vi "Start Stop graph.vi"(8 "error in (no error)":errorcluster, 10 "Start/Stop":bool, 11 "F Generator in":refnum<class "F Generator.lvclass">) -> (0 "error out":errorcluster, 3 "F Generator out":refnum<class "F Generator.lvclass">)   [LabVIEW 2020, in "F Generator.lvlib" / "F Generator.lvclass"]
uses:
  F Generator.lvclass
  F Generator.lvclass/F Generator.ctl
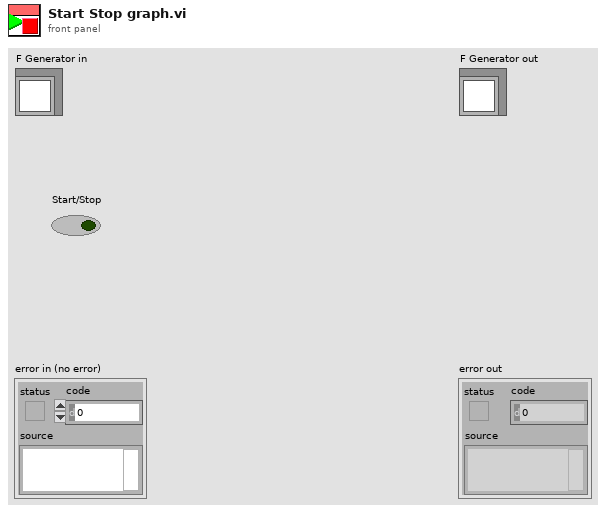
[diagram p1: front panel]
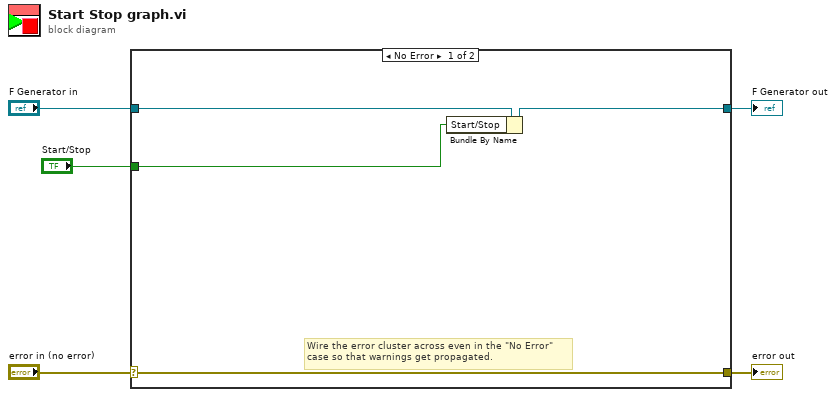
[diagram p0: block diagram]
diagram:
  n1 = case shown="No Error" "error in (no error)" {
    selector: "error in (no error)" -> [w8 w11]
    tunnel: [w8 w11] -> w4
    tunnel: [w7 w10] -> w2
    tunnel: "F Generator in" -> [w9 w10]
    tunnel: "Start/Stop" -> [w6 _]
    frame No Error {
      # "Wire the error cluster across even in the \"No Error\"\ncase so that warnings get propagated."
      n2 = Bundle By Name(cluster=w9, "Start/Stop"=w6) -> (w7:refnum<class "F Generator.lvclass">)
    }
    frame Error {
    }
  }
  "error out" <- w4
  "F Generator out" <- w2
